vi "Interpret Driver Controls.vi"() -> ()   [LabVIEW 2018]
uses:
  <vilib>/Rock Robotics/WPI/DriverStation/WPI_DriverStationDerivedRobotMode.ctl
  Robot Global Data.vi
  SubSystems/Controllers/Driver Controller/Driver Controller Global.vi
  SubSystems/Drive Train/Drive Train Global.vi
  SubSystems/Lift/Lift Global.vi
  <vilib>/addons/control/pid/pid.llb/PID (DBL).vi
  SubSystems/Controllers/Manipulator Controlller/Manipulator Controller Global.vi
  SubSystems/HAB Climber/HAB Climber Global.vi
  SubSystems/Hatch Panel Intake/Hatch Panel Intake Global.vi
  SubSystems/Cargo Intake/Cargo Intake Global.vi
  <vilib>/addons/control/pid/NI_PID_pid.lvlib
panel:
  in  "Last Move Deadband":u32=500
  in  "Last Time Auto":u32=1171826
  in  "Camera Tracking":T1={"proportional gain (Kc)"=0.06, "integral time (Ti, min)"=0.0, "derivative time (Td, min)"=0.0}
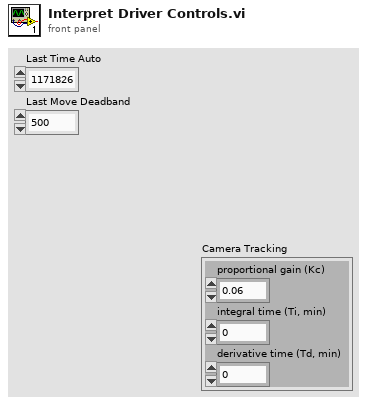
[diagram p1: front panel]
types:
  T1 = cluster{"proportional gain (Kc)":dbl, "integral time (Ti, min)":dbl, "derivative time (Td, min)":dbl}
  T2 = enum16{"Manual", "Hatch Panel Zone 1", "Hatch Panel Zone 2", "Hatch Panel Zone 3", "Cargo Zone 1", "Cargo Zone 2", "Cargo Zone 3", "Cargo Ship Zone"}
  T3 = cluster{"Rollover":dbl, "Yaw":dbl, "Cont Yaw":dbl}
  T4 = typedef "WPI_DriverStationDerivedRobotMode.ctl" = enum16{"Init", "Execute", "Stop"}
  T5 = enum16{"Hatch Panel Zone 1", "Hatch Panel Zone 2", "Hatch Panel Zone 3", "Cargo Zone 1", "Cargo Zone 2", "Cargo Zone 3", "Cargo Ship Zone"}
  T6 = cluster{"offsetAngle H":dbl, "offsetAngle V":dbl, "area":dbl, "skew":dbl, "validTarget":dbl, "latency":dbl}
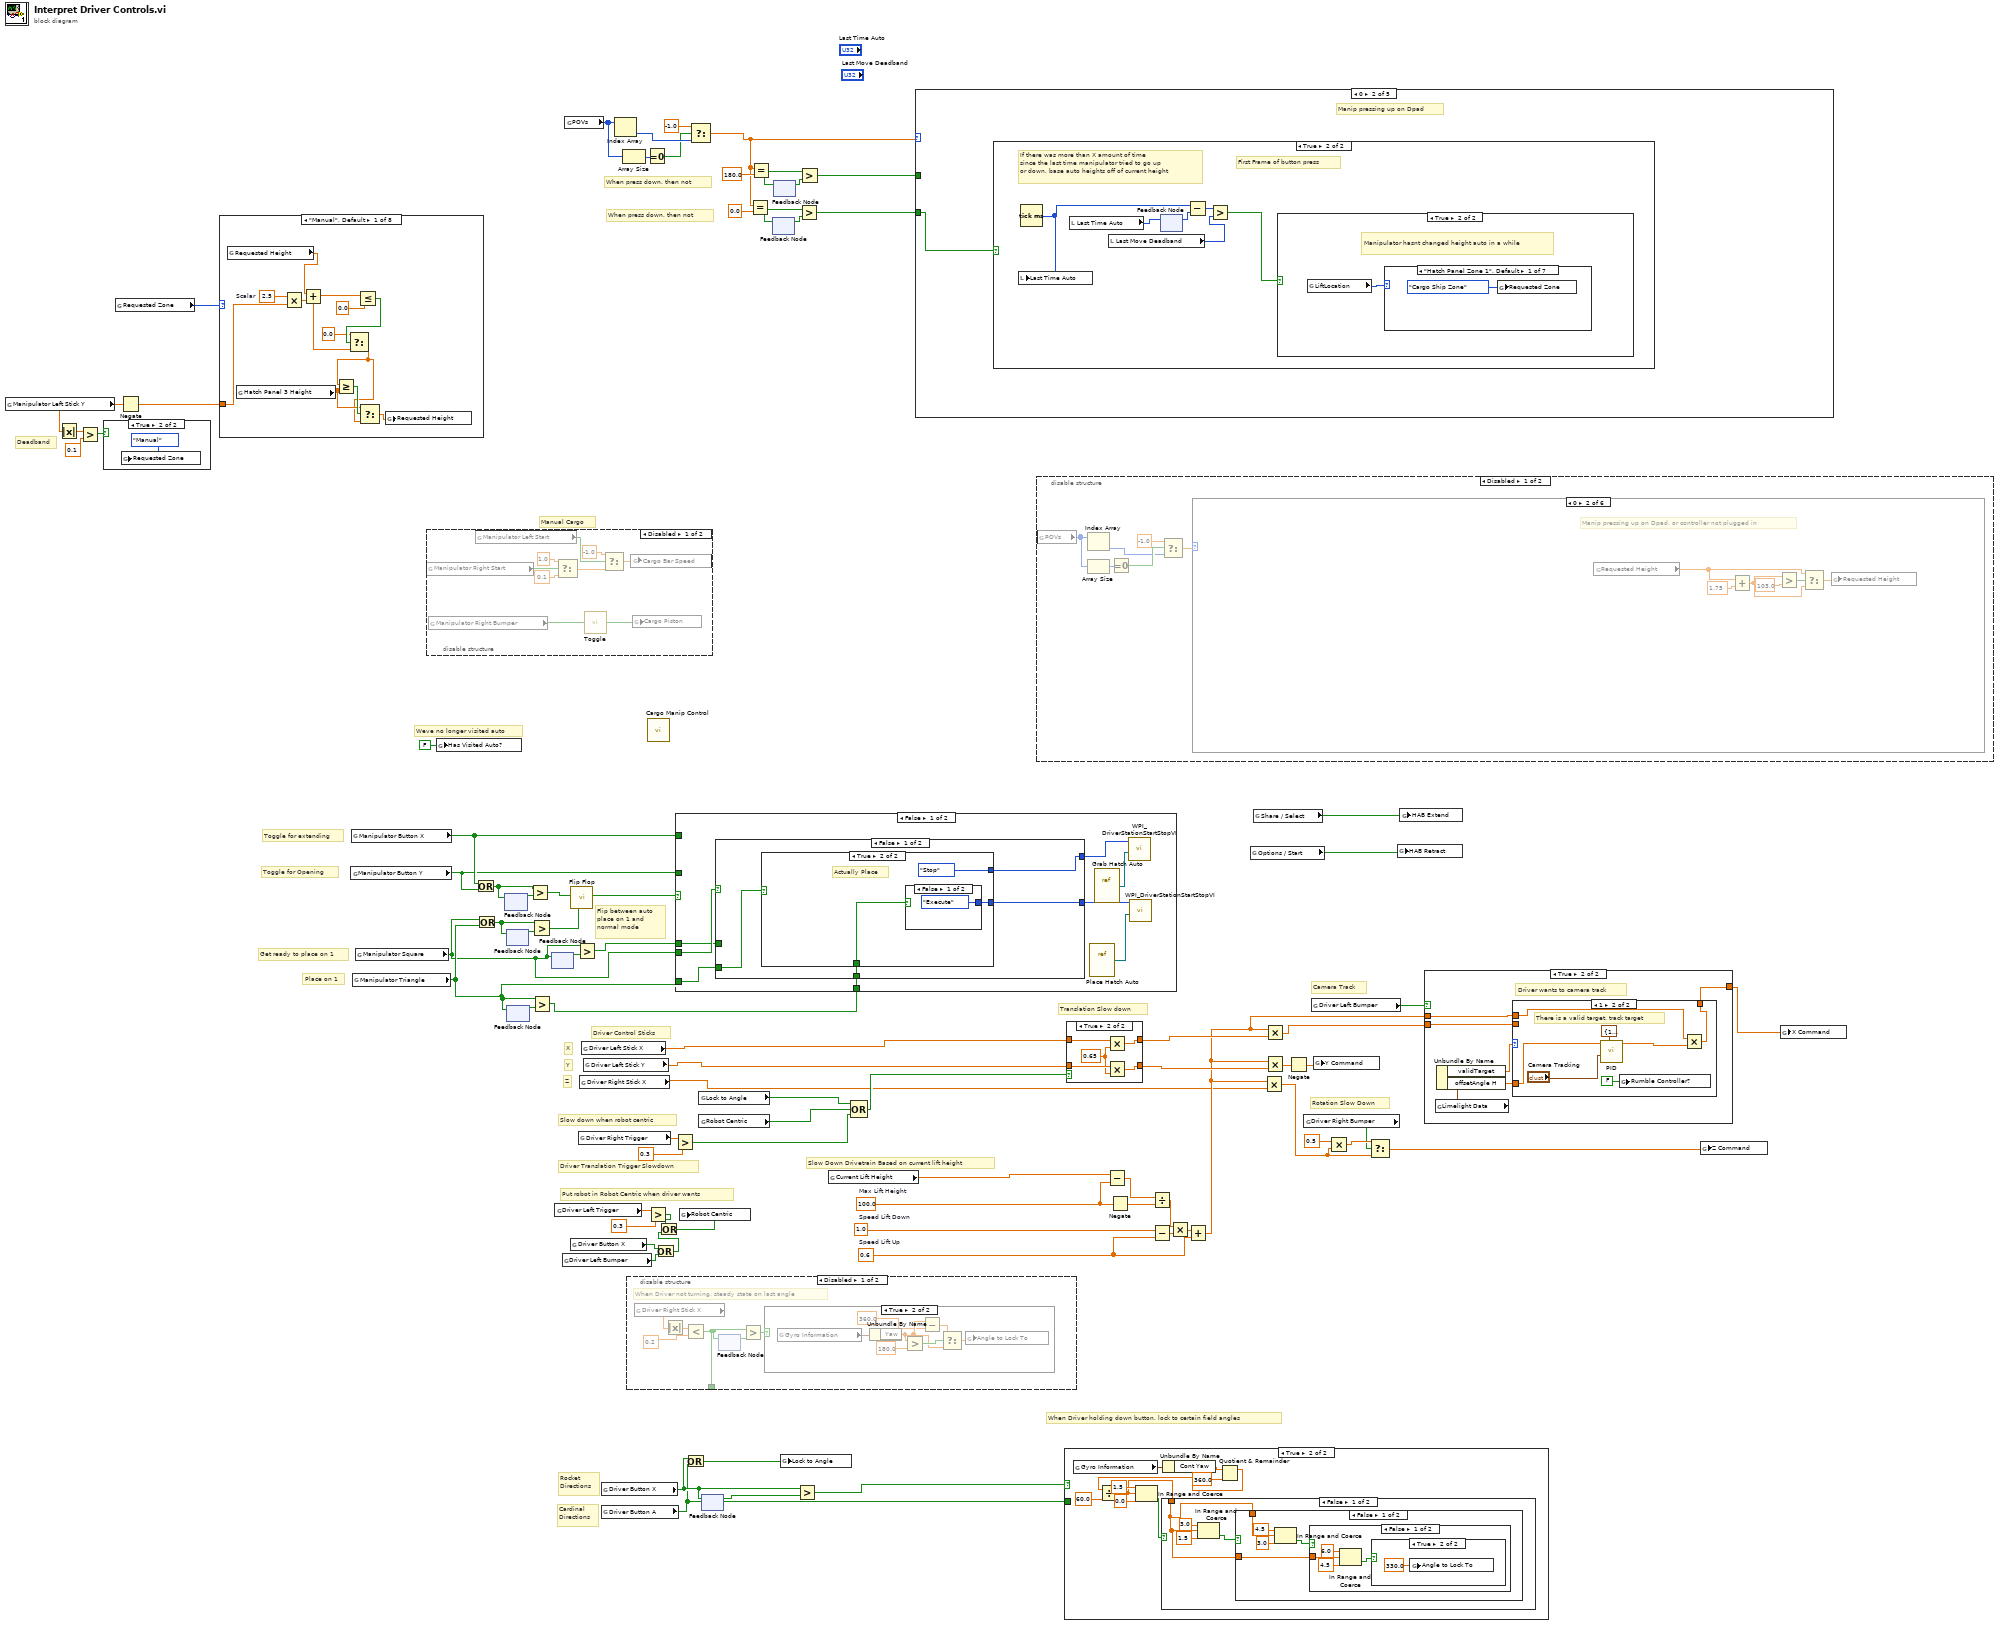
[diagram p0: block diagram]
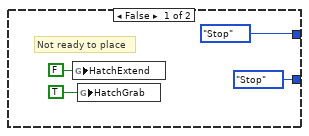
[diagram p2: hidden frame]
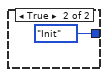
[diagram p3: hidden frame]
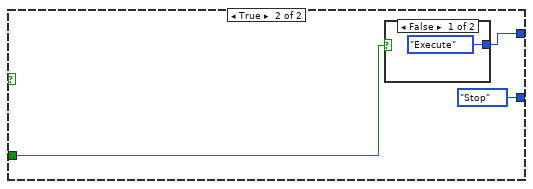
[diagram p4: hidden frame]
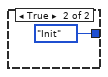
[diagram p5: hidden frame]
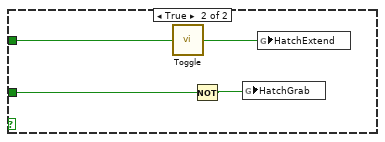
[diagram p6: hidden frame]
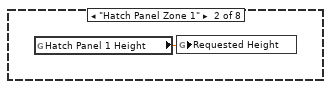
[diagram p8: hidden frame]
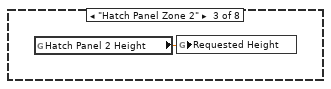
[diagram p9: hidden frame]
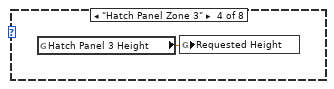
[diagram p10: hidden frame]
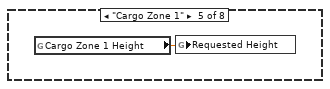
[diagram p11: hidden frame]
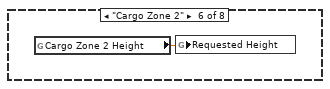
[diagram p12: hidden frame]
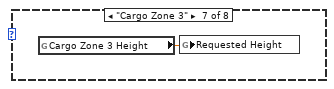
[diagram p13: hidden frame]
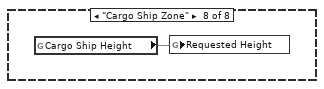
[diagram p14: hidden frame]
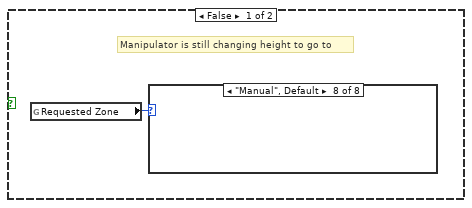
[diagram p17: hidden frame]
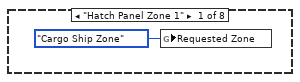
[diagram p18: hidden frame]
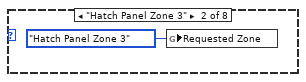
[diagram p19: hidden frame]
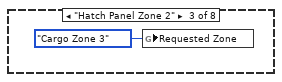
[diagram p20: hidden frame]
diagram:
  w62 = 0.6  # Speed Lift Up
  w66 = 1.0  # Speed Lift Down
  w60 = 100.0  # Max Lift Height
  # "Toggle for Opening"
  # "Toggle for extending"
  # "Place on 1"
  # "Get ready to place on 1"
  # "Flip between auto\nplace on 1 and \nnormal mode"
  # "When press down, then not"
  # "When press down, then not"
  # "Deadband"
  # "Manual Cargo"
  # "Weve no longer visited auto"
  # "Camera Track"
  # "Rotation Slow Down"
  # "Rocket\nDirections"
  # "Cardinal\nDirections"
  # "When Driver holding down button, lock to certain field angles"
  # "Slow Down Drivetrain Based on current lift height"
  # "Put robot in Robot Centric when driver wants"
  # "Slow down when robot centric"
  # "Driver Translation Trigger Slowdown"
  # "Translation Slow down"
  # "Z"
  # "Y"
  # "X"
  # "Driver Control Sticks"
  n1 = global read "Manipulator Controller Global.vi" "Manipulator Left Stick Y"() -> (w31:dbl)
  n2 = Absolute Value(x=w31) -> (abs(x)=w34:dbl)
  n3 = Greater?(x=w34, y=0.1) -> (0:w32:bool)
  n4 = case shown="True" w32 {
    frame False {
    }
    frame True {
      n5 = global write "Lift Global.vi" "Requested Zone"(T2."Manual" ("Requested Zone")) -> ()
    }
  }
  n6 = global read "Lift Global.vi" "Requested Zone"() -> (w35:T2)
  n7 = Negate(x=w31) -> (-x=w30:dbl)
  n8 = case shown="\"Manual\", Default" w35 {
    tunnel: w30 -> [w92 _ _ _ _ _ _ _]
    frame "Manual", Default {
      w91 = 2.5  # Scalar
      n9 = global read "Lift Global.vi" "Requested Height"() -> (w94:dbl)
      n10 = global read "Lift Global.vi" "Hatch Panel 3 Height"() -> (w85:dbl)
      n11 = Multiply(x=w91, y=w92) -> (x*y=w93:dbl)
      n12 = Add(x=w94, y=w93) -> (x+y=w87:dbl)
      n13 = Less Or Equal?(x=w87, y=0.0) -> (x <= y?=w89:bool)
      n14 = Select(t=0.0, s=w89, f=w87) -> (s? t:f=w84:dbl)
      n15 = Greater Or Equal?(x=w84, y=w85) -> (x >= y?=w86:bool)
      n16 = Select(t=w85, s=w86, f=w84) -> (s? t:f=w83:dbl)
      n17 = global write "Lift Global.vi" "Requested Height"(w83) -> ()
    }
    frame "Hatch Panel Zone 1" {
      n18 = global read "Lift Global.vi" "Hatch Panel 1 Height"() -> (w95:dbl)
      n19 = global write "Lift Global.vi" "Requested Height"(w95) -> ()
    }
    frame "Hatch Panel Zone 2" {
      n20 = global read "Lift Global.vi" "Hatch Panel 2 Height"() -> (w96:dbl)
      n21 = global write "Lift Global.vi" "Requested Height"(w96) -> ()
    }
    frame "Hatch Panel Zone 3" {
      n22 = global read "Lift Global.vi" "Hatch Panel 3 Height"() -> (w97:dbl)
      n23 = global write "Lift Global.vi" "Requested Height"(w97) -> ()
    }
    frame "Cargo Zone 1" {
      n24 = global read "Lift Global.vi" "Cargo Zone 1 Height"() -> (w98:dbl)
      n25 = global write "Lift Global.vi" "Requested Height"(w98) -> ()
    }
    frame "Cargo Zone 2" {
      n26 = global read "Lift Global.vi" "Cargo Zone 2 Height"() -> (w99:dbl)
      n27 = global write "Lift Global.vi" "Requested Height"(w99) -> ()
    }
    frame "Cargo Zone 3" {
      n28 = global read "Lift Global.vi" "Cargo Zone 3 Height"() -> (w100:dbl)
      n29 = global write "Lift Global.vi" "Requested Height"(w100) -> ()
    }
    frame "Cargo Ship Zone" {
      n30 = global read "Lift Global.vi" "Cargo Ship Height"() -> (w101:dbl)
      n31 = global write "Lift Global.vi" "Requested Height"(w101) -> ()
    }
  }
  n32 = global read "Manipulator Controller Global.vi" "Manipulator Button Y"() -> (w17:bool)
  n33 = global read "Manipulator Controller Global.vi" "Manipulator Button X"() -> (w18:bool)
  n34 = global read "Manipulator Controller Global.vi" "Manipulator Triangle"() -> (w7:bool)
  n35 = global read "Manipulator Controller Global.vi" "Manipulator Square"() -> (w2:bool)
  n36 = disable-structure shown="Disabled" {
    frame Disabled {
      n37 = global read "Manipulator Controller Global.vi" "Manipulator Right Start"() -> (w107:bool)
      n38 = global read "Manipulator Controller Global.vi" "Manipulator Right Bumper"() -> (w110:bool)
      n39 = global read "Manipulator Controller Global.vi" "Manipulator Left Start"() -> (w106:bool)
      n40 = Select(t=1.0, s=w107, f=0.1) -> (s? t:f=w105:dbl)
      n41 = call "Toggle.vi"("Input"=w110) -> ("Output"=w109:bool)
      n42 = Select(t=-1.0, s=w106, f=w105) -> (s? t:f=w108:dbl)
      n43 = global write "Cargo Intake Global.vi" "Cargo Bar Speed"(w108) -> ()
      n44 = global write "Cargo Intake Global.vi" "Cargo Piston"(w109) -> ()
    }
    frame Enabled {
    }
  }
  n45 = global write "Robot Global Data.vi" "Has Visited Auto?"(FALSE ("Has Visited Auto?")) -> ()
  n46 = Or(x=w18, y=w17) -> (x .or. y?=w15:bool)
  n47 = Or(x=w2, y=w7) -> (x .or. y?=w12:bool)
  n48 = feedback-in #1(w15) -> ()
  n49 = feedback #1() -> (w16:bool)  [unwired: 1 in]
  n50 = feedback #2() -> (w13:bool)  [unwired: 1 in]
  n51 = feedback-in #2(w12) -> ()
  n52 = feedback #3() -> (w9:bool)  [unwired: 1 in]
  n53 = feedback-in #3(w7) -> ()
  n54 = Greater?(x=w15, y=w16) -> (0:w14:bool)
  n55 = Greater?(x=w12, y=w13) -> (0:w11:bool)
  n56 = Greater?(x=w7, y=w9) -> (0:w8:bool)
  n57 = feedback #4() -> (w3:bool)  [unwired: 1 in]
  n58 = feedback-in #4(w2) -> ()
  n59 = global read "Driver Controller Global.vi" "Driver Left Trigger"() -> (w78:dbl)
  n60 = global read "Driver Controller Global.vi" "Driver Left Bumper"() -> (w45:bool)
  n61 = global read "Manipulator Controller Global.vi" "POVs"() -> (w39:i16[])
  n62 = call "Flip Flop.vi"("Line 2"=w11, "Line 1"=w14) -> ("Switch"=w10:bool)  [unwired: 9 in]
  n63 = global read "Driver Controller Global.vi" "Driver Button X"() -> (w46:bool)
  n64 = Greater?(x=w2, y=w3) -> (0:w1:bool)
  n65 = global read "Driver Controller Global.vi" "Driver Right Trigger"() -> (w81:dbl)
  n66 = global read "Driver Controller Global.vi" "Driver Right Stick X"() -> (w4:dbl)
  n67 = global read "Driver Controller Global.vi" "Driver Left Stick X"() -> (w6:dbl)
  n68 = global read "Driver Controller Global.vi" "Driver Left Stick Y"() -> (w5:dbl)
  n69 = global read "Driver Controller Global.vi" "Driver Button X"() -> (w58:bool)
  n70 = global read "Driver Controller Global.vi" "Driver Button A"() -> (w56:bool)
  n71 = Index Array(array=w39) -> (element=w36:i16)  [unwired: 1 in]
  n72 = Array Size(array=w39) -> (size(s)=w38:i32)
  n73 = disable-structure shown="Disabled" {
    disable-tunnel: [w111 _] -> _
    frame Disabled {
      # "When Driver not turning, steady state on last angle"
      n74 = global read "Driver Controller Global.vi" "Driver Right Stick X"() -> (w112:dbl)
      n75 = Absolute Value(x=w112) -> (abs(x)=w116:dbl)
      n76 = Less?(x=w116, y=0.2) -> (x < y?=w111:bool)
      n77 = feedback #5() -> (w114:bool)  [unwired: 1 in]
      n78 = feedback-in #5(w111) -> ()
      n79 = Greater?(x=w111, y=w114) -> (0:w113:bool)
      n80 = case shown="True" w113 {
        frame False {
        }
        frame True {
          n81 = global read "Drive Train Global.vi" "Gyro Information"() -> (w123:T3)
          n82 = Unbundle By Name(w123) -> ("Yaw"=w120:dbl)
          n83 = Greater?(x=w120, y=180.0) -> (0:w121:bool)
          n84 = Subtract(x=w120, y=360.0) -> (x-y=w118:dbl)
          n85 = Select(t=w118, s=w121, f=w120) -> (s? t:f=w117:dbl)
          n86 = global write "Drive Train Global.vi" "Angle to Lock To"(w117) -> ()
        }
      }
    }
    frame Enabled {
    }
  }
  n87 = Equal To 0?(x=w38) -> (x = 0?=w29:bool)
  n88 = call "Cargo Manip Control.vi"() -> ()  [unwired: 12 in]
  n89 = Greater?(x=w78, y=0.3) -> (0:w54:bool)
  n90 = Or(x=w46, y=w45) -> (x .or. y?=w47:bool)
  n91 = Or(x=w54, y=w47) -> (x .or. y?=w52:bool)
  n92 = Greater?(x=w81, y=0.3) -> (0:w73:bool)
  n93 = case shown="False" w10 {
    tunnel: w17 -> [_ w151]
    tunnel: w18 -> [_ w152]
    tunnel: w2 -> [w131 _]
    tunnel: w8 -> [w128 _]
    tunnel: w7 -> [w127 _]
    tunnel: w1 -> [w124 _]
    frame False {
      n94 = case shown="False" w131 {
        tunnel: [w135 WPI_DriverStationDerivedRobotMode."Stop" ("Call Context")] -> w129
        tunnel: w128 -> [w134 _]
        tunnel: w127 -> [w133 _]
        tunnel: [w132 w146] -> w125
        tunnel: w124 -> [_ w145]
        frame False {
          n95 = case shown="True" w133 {
            tunnel: [WPI_DriverStationDerivedRobotMode."Stop" ("Call Context") w142] -> w135
            tunnel: w134 -> [_ w141]
            tunnel: [WPI_DriverStationDerivedRobotMode."Stop" ("Call Context") WPI_DriverStationDerivedRobotMode."Stop" ("Call Context")] -> w132
            frame False {
              # "Not ready to place"
              n96 = global write "Hatch Panel Intake Global.vi" "HatchExtend"(FALSE ("HatchExtend")) -> ()
              n97 = global write "Hatch Panel Intake Global.vi" "HatchGrab"(TRUE ("HatchExtend")) -> ()
            }
            frame True {
              # "Actually Place"
              n98 = case shown="False" w141 {
                tunnel: [WPI_DriverStationDerivedRobotMode."Execute" ("Call Context") WPI_DriverStationDerivedRobotMode."Init" ("Call Context")] -> w142
                frame False {
                }
                frame True {
                }
              }
            }
          }
        }
        frame True {
          n99 = case shown="False" w145 {
            tunnel: [WPI_DriverStationDerivedRobotMode."Execute" ("Call Context") WPI_DriverStationDerivedRobotMode."Init" ("Call Context")] -> w146
            frame False {
            }
            frame True {
            }
          }
        }
      }
      n100 = vi-ref "Place Hatch Auto.vi"() -> (w130:refnum<vi>)
      n101 = vi-ref "Grab Hatch Auto.vi"() -> (w126:refnum<vi>)
      n102 = call <vilib>:"WPI_DriverStationStartStopVI.vi"("VI in"=w126, "Call Context"=w125) -> ()  [unwired: 10 in]
      n103 = call <vilib>:"WPI_DriverStationStartStopVI.vi"("VI in"=w130, "Call Context"=w129) -> ()  [unwired: 10 in]
    }
    frame True {
      n104 = call "Toggle.vi"("Input"=w152) -> ("Output"=w153:bool)
      n105 = Not(x=w151) -> (.not. x?=w150:bool)
      n106 = global write "Hatch Panel Intake Global.vi" "HatchGrab"(w150) -> ()
      n107 = global write "Hatch Panel Intake Global.vi" "HatchExtend"(w153) -> ()
    }
  }
  n108 = global write "Drive Train Global.vi" "Robot Centric"(w52) -> ()
  n109 = Or(x=w58, y=w56) -> (x .or. y?=w55:bool)
  n110 = Select(t=-1.0, s=w29, f=w36) -> (s? t:f=w21:dbl)
  n111 = global read "Drive Train Global.vi" "Lock to Angle"() -> (w53:bool)
  n112 = global read "Drive Train Global.vi" "Robot Centric"() -> (w72:bool)
  n113 = feedback #6() -> (w59:bool)  [unwired: 1 in]
  n114 = feedback-in #6(w58) -> ()
  n115 = Equal?(x=w21, y=0.0) -> (x = y?=w24:bool)
  n116 = Equal?(x=w21, y=180.0) -> (x = y?=w26:bool)
  n117 = feedback #7() -> (w23:bool)  [unwired: 1 in]
  n118 = feedback-in #7(w24) -> ()
  n119 = feedback-in #8(w26) -> ()
  n120 = feedback #8() -> (w27:bool)  [unwired: 1 in]
  n121 = global write "Drive Train Global.vi" "Lock to Angle"(w55) -> ()
  n122 = Greater?(x=w58, y=w59) -> (0:w57:bool)
  n123 = Greater?(x=w24, y=w23) -> (0:w20:bool)
  n124 = Greater?(x=w26, y=w27) -> (0:w25:bool)
  n125 = global read "Lift Global.vi" "Current Lift Height"() -> (w68:dbl)
  n126 = Compound Arithmetic op=OR(w53, w72, w73) -> (w71:bool)
  n127 = case shown="0" w21 {
    tunnel: w25 -> [_ _ w177 _ _]
    tunnel: w20 -> [_ w154 _ _ _]
    frame -1, Default {
      # "Nothing on the D-Pad is pressed!"
    }
    frame 0 {
      # "Manip pressing up on Dpad"
      n128 = case shown="True" w154 {
        frame False {
          # "Still pressing button, do nothing"
        }
        frame True {
          # "First Frame of button press"
          # "If there was more than X amount of time\nsince the last time manipulator tried to go up\nor down, base auto heights off of current height"
          n129 = Tick Count (ms)() -> (millisecond timer value=w157:u32)
          n130 = local write "Last Time Auto"(w157) -> ()
          n131 = local read "Last Time Auto"() -> (w156:u32)
          n132 = local read "Last Move Deadband"() -> (w158:u32)
          n133 = feedback #9() -> (w155:u32)  [unwired: 1 in]
          n134 = feedback-in #9(w156) -> ()
          n135 = Subtract(x=w157, y=w155) -> (x-y=w160:u32)
          n136 = Greater?(x=w160, y=w158) -> (0:w159:bool)
          n137 = case shown="True" w159 {
            frame False {
              # "Manipulator is still changing height to go to"
              n138 = global read "Lift Global.vi" "Requested Zone"() -> (w161:T2)
              n139 = case shown="\"Manual\", Default" w161 {
                frame "Hatch Panel Zone 1" {
                  n140 = global write "Lift Global.vi" "Requested Zone"(T2."Cargo Ship Zone" ("Requested Zone")) -> ()
                }
                frame "Hatch Panel Zone 3" {
                  n141 = global write "Lift Global.vi" "Requested Zone"(T2."Hatch Panel Zone 3" ("Requested Zone")) -> ()
                }
                frame "Hatch Panel Zone 2" {
                  n142 = global write "Lift Global.vi" "Requested Zone"(T2."Cargo Zone 3" ("Requested Zone")) -> ()
                }
                frame "Cargo Zone 1" {
                  n143 = global write "Lift Global.vi" "Requested Zone"(T2."Hatch Panel Zone 1" ("Requested Zone")) -> ()
                }
                frame "Cargo Zone 2" {
                  n144 = global write "Lift Global.vi" "Requested Zone"(T2."Hatch Panel Zone 2" ("Requested Zone")) -> ()
                }
                frame "Cargo Zone 3" {
                  n145 = global write "Lift Global.vi" "Requested Zone"(T2."Hatch Panel Zone 3" ("Requested Zone")) -> ()
                }
                frame "Cargo Ship Zone" {
                  n146 = global write "Lift Global.vi" "Requested Zone"(T2."Cargo Zone 2" ("Requested Zone")) -> ()
                }
                frame "Manual", Default {
                }
              }
            }
            frame True {
              # "Manipulator hasnt changed height auto in a while"
              n147 = global read "Lift Global.vi" "LiftLocation"() -> (w169:T5)
              n148 = case shown="\"Hatch Panel Zone 1\", Default" w169 {
                frame "Hatch Panel Zone 1", Default {
                  n149 = global write "Lift Global.vi" "Requested Zone"(T2."Cargo Ship Zone" ("Requested Zone")) -> ()
                }
                frame "Hatch Panel Zone 3" {
                  n150 = global write "Lift Global.vi" "Requested Zone"(T2."Hatch Panel Zone 3" ("Requested Zone")) -> ()
                }
                frame "Hatch Panel Zone 2" {
                  n151 = global write "Lift Global.vi" "Requested Zone"(T2."Cargo Zone 3" ("Requested Zone")) -> ()
                }
                frame "Cargo Zone 1" {
                  n152 = global write "Lift Global.vi" "Requested Zone"(T2."Hatch Panel Zone 1" ("Requested Zone")) -> ()
                }
                frame "Cargo Zone 2" {
                  n153 = global write "Lift Global.vi" "Requested Zone"(T2."Hatch Panel Zone 2" ("Requested Zone")) -> ()
                }
                frame "Cargo Zone 3" {
                  n154 = global write "Lift Global.vi" "Requested Zone"(T2."Hatch Panel Zone 3" ("Requested Zone")) -> ()
                }
                frame "Cargo Ship Zone" {
                  n155 = global write "Lift Global.vi" "Requested Zone"(T2."Cargo Zone 2" ("Requested Zone")) -> ()
                }
              }
            }
          }
        }
      }
    }
    frame 180 {
      # "Manip pressing down on Dpad"
      n156 = case shown="True" w177 {
        frame False {
          # "Still pressing button, do nothing"
        }
        frame True {
          # "First frame of button press"
          # "If there was more than X amount of time\nsince the last time manipulator tried to go up\nor down, base auto heights off of current height"
          n157 = Tick Count (ms)() -> (millisecond timer value=w182:u32)
          n158 = local write "Last Time Auto"(w182) -> ()
          n159 = local read "Last Time Auto"() -> (w179:u32)
          n160 = local read "Last Move Deadband"() -> (w181:u32)
          n161 = feedback #10() -> (w178:u32)  [unwired: 1 in]
          n162 = feedback-in #10(w179) -> ()
          n163 = Subtract(x=w182, y=w178) -> (x-y=w183:u32)
          n164 = Greater?(x=w183, y=w181) -> (0:w180:bool)
          n165 = case shown="False" w180 {
            frame False {
              # "Manipulator is still changing height to go to"
              n166 = global read "Lift Global.vi" "Requested Zone"() -> (w184:T2)
              n167 = case shown="\"Cargo Ship Zone\"" w184 {
                frame "Hatch Panel Zone 1" {
                  n168 = global write "Lift Global.vi" "Requested Zone"(T2."Cargo Zone 1" ("Requested Zone")) -> ()
                }
                frame "Hatch Panel Zone 3" {
                  n169 = global write "Lift Global.vi" "Requested Zone"(T2."Cargo Zone 3" ("Requested Zone")) -> ()
                }
                frame "Hatch Panel Zone 2" {
                  n170 = global write "Lift Global.vi" "Requested Zone"(T2."Cargo Zone 2" ("Requested Zone")) -> ()
                }
                frame "Cargo Zone 1" {
                  n171 = global write "Lift Global.vi" "Requested Zone"(T2."Cargo Zone 1" ("Requested Zone")) -> ()
                }
                frame "Cargo Zone 2" {
                  n172 = global write "Lift Global.vi" "Requested Zone"(T2."Cargo Ship Zone" ("Requested Zone")) -> ()
                }
                frame "Cargo Zone 3" {
                  n173 = global write "Lift Global.vi" "Requested Zone"(T2."Hatch Panel Zone 2" ("Requested Zone")) -> ()
                }
                frame "Cargo Ship Zone" {
                  n174 = global write "Lift Global.vi" "Requested Zone"(T2."Hatch Panel Zone 1" ("Requested Zone")) -> ()
                }
                frame "Manual", Default {
                }
              }
            }
            frame True {
              # "Manipulator hasnt changed height auto in a while"
              n175 = global read "Lift Global.vi" "LiftLocation"() -> (w192:T5)
              n176 = case shown="\"Hatch Panel Zone 1\", Default" w192 {
                frame "Hatch Panel Zone 1", Default {
                  n177 = global write "Lift Global.vi" "Requested Zone"(T2."Cargo Zone 1" ("Requested Zone")) -> ()
                }
                frame "Hatch Panel Zone 3" {
                  n178 = global write "Lift Global.vi" "Requested Zone"(T2."Cargo Zone 3" ("Requested Zone")) -> ()
                }
                frame "Hatch Panel Zone 2" {
                  n179 = global write "Lift Global.vi" "Requested Zone"(T2."Cargo Zone 2" ("Requested Zone")) -> ()
                }
                frame "Cargo Zone 1" {
                  n180 = global write "Lift Global.vi" "Requested Zone"(T2."Cargo Zone 1" ("Requested Zone")) -> ()
                }
                frame "Cargo Zone 2" {
                  n181 = global write "Lift Global.vi" "Requested Zone"(T2."Cargo Ship Zone" ("Requested Zone")) -> ()
                }
                frame "Cargo Zone 3" {
                  n182 = global write "Lift Global.vi" "Requested Zone"(T2."Hatch Panel Zone 2" ("Requested Zone")) -> ()
                }
                frame "Cargo Ship Zone" {
                  n183 = global write "Lift Global.vi" "Requested Zone"(T2."Hatch Panel Zone 1" ("Requested Zone")) -> ()
                }
              }
            }
          }
        }
      }
    }
    frame 90 {
      # "Go to Cargo in Cargo Ship Height"
      # "Right on D-Pad"
      n184 = global write "Lift Global.vi" "Requested Zone"(T2."Cargo Ship Zone" ("Requested Zone")) -> ()
    }
    frame 270 {
      # "Go to Hatch Level 1 Height"
      # "Left on D-Pad"
      n185 = global write "Lift Global.vi" "Requested Zone"(T2."Hatch Panel Zone 1" ("Requested Zone")) -> ()
    }
  }
  n186 = disable-structure shown="Disabled" {
    frame Disabled {
      n187 = global read "Manipulator Controller Global.vi" "POVs"() -> (w207:i16[])
      n188 = Index Array(array=w207) -> (element=w202:i16)  [unwired: 1 in]
      n189 = Array Size(array=w207) -> (size(s)=w206:i32)
      n190 = Equal To 0?(x=w206) -> (x = 0?=w204:bool)
      n191 = Select(t=-1.0, s=w204, f=w202) -> (s? t:f=w205:dbl)
      n192 = case shown="0" w205 {
        frame -1 {
          # "If the value changed (manip pressed button)\nchange set lift height to match"
          # "When button goes from\nnot pressed to pressed"
          n193 = global read "Manipulator Controller Global.vi" "Manipulator Square"() -> (w213:bool)
          n194 = feedback #11() -> (w214:bool)  [unwired: 1 in]
          n195 = feedback-in #11(w213) -> ()
          n196 = Greater?(x=w213, y=w214) -> (0:w210:bool)
          n197 = feedback #12() -> (w208:dbl)  [unwired: 1 in]
          n198 = feedback #13() -> (w212:dbl)  [unwired: 1 in]
          n199 = case shown="False" w210 {
            tunnel: [w224 w239] -> w209
            tunnel: w212 -> [w225 w238]
            frame False {
              # "When button goes from\nnot pressed to pressed"
              n200 = global read "Manipulator Controller Global.vi" "Manipulator Triangle"() -> (w227:bool)
              n201 = feedback #14() -> (w226:bool)  [unwired: 1 in]
              n202 = feedback-in #14(w227) -> ()
              n203 = Greater?(x=w227, y=w226) -> (0:w223:bool)
              n204 = case shown="True" w223 {
                tunnel: w225 -> [w228 w230]
                tunnel: [w228 w232] -> w224
                frame False {
                }
                frame True {
                  # "If counter smaller than 5\nadd 1"
                  n205 = Less?(x=w230, y=5.0) -> (x < y?=w229:bool)
                  n206 = case shown="True" w229 {
                    tunnel: [w233 w235] -> w232
                    tunnel: w230 -> [w233 w234]
                    frame False {
                    }
                    frame True {
                      n207 = Increment(x=w234) -> (x+1=w235:dbl)
                    }
                  }
                }
              }
            }
            frame True {
              # "If counter bigger than 0\nsubtract 1"
              n208 = Greater?(x=w238, y=0.0) -> (0:w237:bool)
              n209 = case shown="False" w237 {
                tunnel: [0.0 ("y") w242] -> w239
                tunnel: w238 -> [_ w241]
                frame False {
                }
                frame True {
                  n210 = Decrement(x=w241) -> (x-1=w242:dbl)
                }
              }
            }
          }
          n211 = feedback-in #12(w209) -> ()
          n212 = Not Equal?(x=w209, y=w208) -> (x != y?=w211:bool)
          n213 = case shown="True" w211 {
            tunnel: w209 -> [_ w215]
            frame False {
              # "Manipulator didnt request change"
            }
            frame True {
              # "Set height request to new value"
              n214 = case shown="0, Default" w215 {
                tunnel: [w217 w218 w219 w220 w221 w222] -> w216
                frame 0, Default {
                  n215 = global read "Lift Global.vi" "Cargo Zone 1 Height"() -> (w217:dbl)
                }
                frame 1 {
                  n216 = global read "Lift Global.vi" "Hatch Panel 1 Height"() -> (w218:dbl)
                }
                frame 2 {
                  n217 = global read "Lift Global.vi" "Cargo Zone 2 Height"() -> (w219:dbl)
                }
                frame 3 {
                  n218 = global read "Lift Global.vi" "Hatch Panel 2 Height"() -> (w220:dbl)
                }
                frame 4 {
                  n219 = global read "Lift Global.vi" "Cargo Zone 3 Height"() -> (w221:dbl)
                }
                frame 5 {
                  n220 = global read "Lift Global.vi" "Hatch Panel 3 Height"() -> (w222:dbl)
                }
              }
              n221 = global write "Lift Global.vi" "Requested Height"(w216) -> ()
            }
          }
          n222 = global write "Lift Global.vi" "Lift Auto Position"(w209) -> ()
          n223 = feedback-in #13(w209) -> ()
        }
        frame 0 {
          # "Manip pressing up on Dpad, or controller not plugged in"
          n224 = global read "Lift Global.vi" "Requested Height"() -> (w244:dbl)
          n225 = Add(x=w244, y=1.75) -> (x+y=w243:dbl)
          n226 = Greater?(x=w243, y=103.0) -> (0:w245:bool)
          n227 = Select(t=w244, s=w245, f=w243) -> (s? t:f=w246:dbl)
          n228 = global write "Lift Global.vi" "Requested Height"(w246) -> ()
        }
        frame 180 {
          # "Manip pressing down on Dpad"
          n229 = global read "Lift Global.vi" "Requested Height"() -> (w249:dbl)
          n230 = Add(x=w249, y=-1.0) -> (x+y=w251:dbl)
          n231 = Less?(x=w251, y=0.0) -> (x < y?=w252:bool)
          n232 = Select(t=w249, s=w252, f=w251) -> (s? t:f=w250:dbl)
          n233 = global write "Lift Global.vi" "Requested Height"(w250) -> ()
        }
        frame 90 {
          # "Go to Cargo in Cargo Ship Height"
          # "Right on D-Pad"
          n234 = global read "Lift Global.vi" "Cargo Ship Height"() -> (w255:dbl)
          n235 = global write "Lift Global.vi" "Requested Height"(w255) -> ()
        }
        frame 270 {
          # "Go to Hatch Level 1 Height"
          # "Left on D-Pad"
          n236 = global read "Lift Global.vi" "Hatch Panel 1 Height"() -> (w256:dbl)
          n237 = global write "Lift Global.vi" "Requested Height"(w256) -> ()
        }
        frame -100, Default {
        }
      }
    }
    frame Enabled {
    }
  }
  n238 = case shown="True" w57 {
    tunnel: w56 -> [w258 _]
    frame False {
      n239 = feedback #15() -> (w259:bool)  [unwired: 1 in]
      n240 = feedback-in #15(w258) -> ()
      n241 = Greater?(x=w258, y=w259) -> (0:w257:bool)
      n242 = case shown="True" w257 {
        frame False {
        }
        frame True {
          n243 = global read "Drive Train Global.vi" "Gyro Information"() -> (w266:T3)
          n244 = Unbundle By Name(w266) -> ("Yaw"=w263:dbl)
          n245 = Add(x=w263, y=180.0) -> (x+y=w262:dbl)
          n246 = Divide(x=w262, y=90.0) -> (x/y=w264:dbl)
          n247 = Round To Nearest(number=w264) -> (nearest integer value=w260:dbl)
          n248 = case shown="1" w260 {
            frame 0, Default {
              n249 = global write "Drive Train Global.vi" "Angle to Lock To"(180.0 ("Angle to Lock To")) -> ()
            }
            frame 1 {
              n250 = global write "Drive Train Global.vi" "Angle to Lock To"(270.0 ("Angle to Lock To")) -> ()
            }
            frame 2 {
              n251 = global write "Drive Train Global.vi" "Angle to Lock To"(0.0 ("Angle to Lock To")) -> ()
            }
            frame 3 {
              n252 = global write "Drive Train Global.vi" "Angle to Lock To"(90.0 ("Angle to Lock To")) -> ()
            }
            frame 4 {
              n253 = global write "Drive Train Global.vi" "Angle to Lock To"(180.0 ("Angle to Lock To")) -> ()
            }
          }
        }
      }
    }
    frame True {
      n254 = global read "Drive Train Global.vi" "Gyro Information"() -> (w280:T3)
      n255 = Unbundle By Name(w280) -> ("Cont Yaw"=w278:dbl)
      n256 = Quotient & Remainder(x=w278, y=360.0) -> (x-y*floor(x/y)=w276:dbl)  [unwired: 1 out]
      n257 = Divide(x=w276, y=60.0) -> (x/y=w272:dbl)
      n258 = In Range and Coerce(upper limit=1.5, x=w272, lower limit=0.0) -> (In Range?=w273:bool)  [unwired: 1 out]
      n259 = case shown="False" w273 {
        tunnel: w272 -> [w281 _]
        frame False {
          n260 = In Range and Coerce(upper limit=3.0, x=w281, lower limit=1.5) -> (In Range?=w282:bool)  [unwired: 1 out]
          n261 = case shown="False" w282 {
            tunnel: w281 -> [w287 _]
            tunnel: w281 -> [w285 _]
            frame False {
              n262 = In Range and Coerce(upper limit=4.5, x=w287, lower limit=3.0) -> (In Range?=w286:bool)  [unwired: 1 out]
              n263 = case shown="False" w286 {
                tunnel: w285 -> [w291 _]
                frame False {
                  n264 = In Range and Coerce(upper limit=6.0, x=w291, lower limit=4.5) -> (In Range?=w290:bool)  [unwired: 1 out]
                  n265 = case shown="True" w290 {
                    frame False {
                    }
                    frame True {
                      n266 = global write "Drive Train Global.vi" "Angle to Lock To"(330.0 ("Angle to Lock To")) -> ()
                    }
                  }
                }
                frame True {
                  n267 = global write "Drive Train Global.vi" "Angle to Lock To"(210.0 ("Angle to Lock To")) -> ()
                }
              }
            }
            frame True {
              n268 = global write "Drive Train Global.vi" "Angle to Lock To"(150.0 ("Angle to Lock To")) -> ()
            }
          }
        }
        frame True {
          n269 = global write "Drive Train Global.vi" "Angle to Lock To"(30.0 ("Angle to Lock To")) -> ()
        }
      }
    }
  }
  n270 = case shown="True" w71 {
    tunnel: w5 -> [w299 w304]
    tunnel: [w299 w303] -> w70
    tunnel: [w298 w302] -> w69
    tunnel: w6 -> [w298 w301]
    frame False {
    }
    frame True {
      w300 = 0.65 ("Y Slower")
      n271 = Multiply(x=w301, y=w300) -> (x*y=w302:dbl)
      n272 = Multiply(x=w304, y=w300) -> (x*y=w303:dbl)
    }
  }
  n273 = Subtract(x=w68, y=w60) -> (x-y=w67:dbl)
  n274 = Negate(x=w60) -> (-x=w61:dbl)
  n275 = Divide(x=w67, y=w61) -> (x/y=w65:dbl)
  n276 = Subtract(x=w66, y=w62) -> (x-y=w64:dbl)
  n277 = Multiply(x=w65, y=w64) -> (x*y=w63:dbl)
  n278 = Add(x=w63, y=w62) -> (x+y=w19:dbl)
  n279 = global read "Manipulator Controller Global.vi" "Options / Start"() -> (w43:bool)
  n280 = global read "Manipulator Controller Global.vi" "Share / Select"() -> (w44:bool)
  n281 = Multiply(x=w19, y=w4) -> (x*y=w77:dbl)
  n282 = Multiply(x=w19, y=w69) -> (x*y=w49:dbl)
  n283 = Multiply(x=w19, y=w70) -> (x*y=w42:dbl)
  n284 = Negate(x=w42) -> (-x=w41:dbl)
  n285 = global read "Driver Controller Global.vi" "Driver Right Bumper"() -> (w74:bool)
  n286 = global read "Driver Controller Global.vi" "Driver Left Bumper"() -> (w51:bool)
  n287 = global write "Drive Train Global.vi" "Y Command"(w41) -> ()
  n288 = Multiply(x=0.5, y=w77) -> (x*y=w76:dbl)
  n289 = Select(t=w76, s=w74, f=w77) -> (s? t:f=w50:dbl)
  n290 = global write "HAB Climber Global.vi" "HAB Retract"(w43) -> ()
  n291 = global write "HAB Climber Global.vi" "HAB Extend"(w44) -> ()
  n292 = case shown="True" w51 {
    tunnel: w49 -> [w306 w310]
    tunnel: [w306 w308] -> w48
    tunnel: w19 -> [_ w307]
    frame False {
      # "Driver not attepting to camera track, be normal"
      n293 = global write "Driver Controller Global.vi" "Rumble Controller?"(FALSE ("Rumble Controller?")) -> ()
    }
    frame True {
      # "Driver wants to camera track"
      n294 = global read "Robot Global Data.vi" "Limelight Data"() -> (w312:T6)
      n295 = Unbundle By Name(w312) -> ("validTarget"=w311:dbl, "offsetAngle H"=w309:dbl)
      n296 = case shown="1" w311 {
        tunnel: w310 -> [w313 _]
        tunnel: w309 -> [_ w318]
        tunnel: [w313 w317] -> w308
        tunnel: w307 -> [_ w315]
        frame 0, Default {
          # "No Valid Target, keep using driver controls\nand rumble controller so knows not tracking"
          n297 = global write "Driver Controller Global.vi" "Rumble Controller?"(TRUE ("Rumble Controller?")) -> ()
        }
        frame 1 {
          # "There is a valid target, track target"
          n298 = call-poly <vilib>:"PID.vi"("output range"=cluster{"output high":dbl, "output low":dbl} {"output high"=1.0, "output low"=-1.0}, "PID gains"="Camera Tracking", "setpoint"=w318) -> ("output"=w316:dbl)  [unwired: 7 in, 1 out]
          n299 = global write "Driver Controller Global.vi" "Rumble Controller?"(FALSE ("Rumble Controller?")) -> ()
          n300 = Multiply(x=w315, y=w316) -> (x*y=w317:dbl)
        }
      }
    }
  }
  n301 = global write "Drive Train Global.vi" "Z Command"(w50) -> ()
  n302 = global write "Drive Train Global.vi" "X Command"(w48) -> ()
